vi "rot3.vi"(4 "y":dbl, 6 "FB_In":cluster{timestamp[], dbl[]}) -> (0 "XY_Graph":cluster{dbl[], dbl[]}, 2 "FB_Out":cluster{timestamp[], dbl[]}, 3 "current time":timestamp)   [LabVIEW 2010]
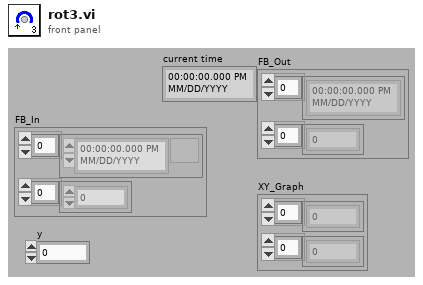
[diagram p1: front panel]
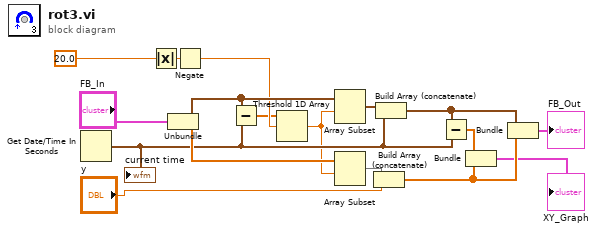
[diagram p0: block diagram]
diagram:
  n1 = Get Date/Time In Seconds() -> (seconds since 1Jan1904=w9:timestamp)
  "current time" <- w9
  n2 = Absolute Value(x=20.0 ("Duration")) -> (abs(x)=w10:dbl)
  n3 = Unbundle("FB_In") -> (w14:timestamp[], w15:dbl[])
  n4 = Negate(x=w10) -> (-x=w11:dbl)
  n5 = Subtract(x=w14, y=w9) -> (x-y=w4:dbl[])
  n6 = Threshold 1D Array(2:w11, 3:w4) -> (0:w2:dbl)  [unwired: 1 in]
  n7 = Array Subset(array=w14, index=w2) -> (w3:timestamp[])  [unwired: 1 in]
  n8 = Array Subset(array=w15, index=w2) -> (w1:dbl[])  [unwired: 1 in]
  n9 = Build Array (concatenate)(w1, "y") -> (w12:dbl[])
  n10 = Build Array (concatenate)(w3, w9) -> (w13:timestamp[])
  n11 = Subtract(x=w13, y=w9) -> (x-y=w8:dbl[])
  n12 = Bundle(w8, w12) -> (→"XY_Graph":cluster{dbl[], dbl[]})  [unwired: 1 in]
  n13 = Bundle(w13, w12) -> (→"FB_Out":cluster{timestamp[], dbl[]})  [unwired: 1 in]
